vi "设备状态循环显示.vi"(7 "cmd:":string, 9 "Str引用句柄":refnum<vi>, 10 "新信息输入":string) -> ()   [LabVIEW 2017]
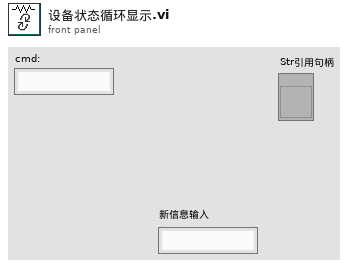
[diagram p1: front panel]
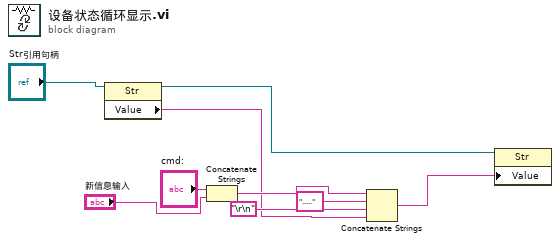
[diagram p0: block diagram]
diagram:
  n1 = property class="Str"(reference="Str引用句柄") -> (reference out=w2:refnum<vi>, "Value"=w1:string)  [unwired: 1 in, 1 out]
  n2 = Concatenate Strings("cmd:", "新信息输入") -> (w5:string)
  n3 = Concatenate Strings(w5, "....." ("字符串"), "\r\n", w1) -> (w4:string)
  n4 = property class="Str"(reference=w2, "Value"=w4) -> ()  [unwired: 1 in, 2 out]
